vi "WriteBufferError.vi"(8 "error in (no error)":errorcluster, 11 "buffer-errors":T1 items=["No error"=0, "Generic Buffer error"=548500, "Generic Custom Buffer error"=548600, "Buffer is full"=548501, "Buffer is empty"=548502, "Buffer size cannot be 0"=548503, "Buffer reference is invalid"=548504, "Buffer event reference invalid"=548505, "Buffer Type not supported"=548506, "Not enough space in the buffer for this operation"=548507]) -> (0 "error out":errorcluster)   [LabVIEW 2013, in "CircularBuffer.lvlib" / "VariantBuffer.lvclass"]
uses:
  VariantBuffer.lvclass
  buffer-errors -- ring.ctl
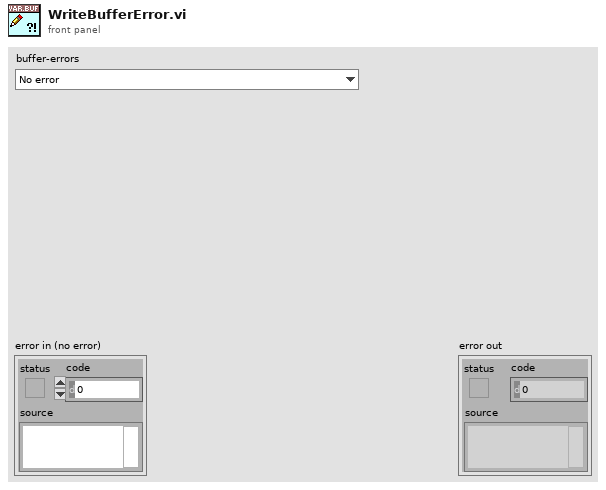
[diagram p1: front panel]
types:
  T1 = typedef "CircularBuffer.lvlib/VariantBuffer.lvclass/buffer-errors -- ring.ctl" = i32
  T2 = typedef "LVStringsAndValuesArrayTypeDef_I32.ctl" = cluster{"String":string, "Value":i32}[]
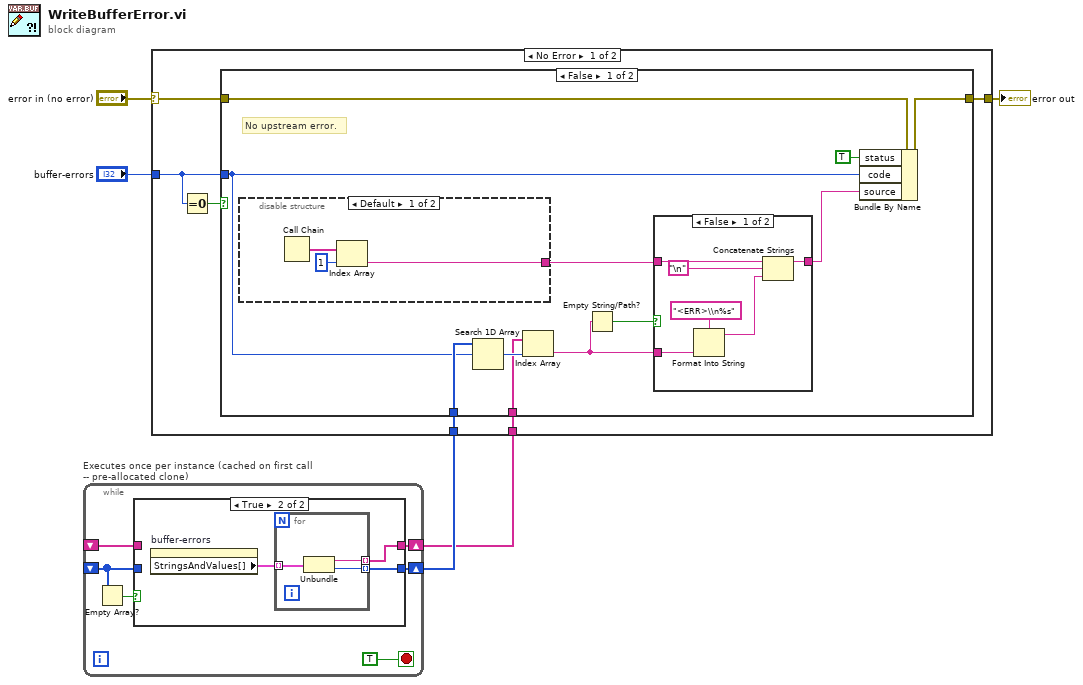
[diagram p0: block diagram]
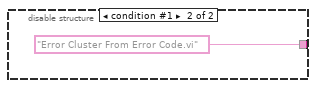
[diagram p4: hidden frame]
diagram:
  n1 = while "Executes once per instance (cached on first call -- pre-allocated clone)" {
    shift-right: [w11] -> w2
    shift-left: _ -> [w6]
    shift-right: [w10] -> w1
    shift-left: _ -> [w8]
    stop <- TRUE stop-if-true
    n2 = Empty Array?(array=w6) -> (empty?=w7:bool)
    n3 = case shown="True" w7 {
      tunnel: [w12 w15] -> w11
      tunnel: [w13 w14] -> w10
      tunnel: w6 -> [w12 _]
      tunnel: w8 -> [w13 _]
      frame False {
      }
      frame True {
        n4 = property on="buffer-errors" class="Ring (strict)"() -> ("StringsAndValues[]"=w16:T2)  [unwired: 2 in, 2 out]
        n5 = for {
          tunnel: w16 -> [w19] mode=indexing
          tunnel: [w18] -> w14 mode=indexing
          tunnel: [w17] -> w15 mode=indexing
          n6 = Unbundle(w19) -> ("String"=w18:string, "Value"=w17:i32)
        }
      }
    }
  }
  n7 = case shown="No Error" "error in (no error)" {
    selector: "error in (no error)" -> [w22 w49]
    tunnel: [w25 w49] -> w5
    tunnel: "buffer-errors" -> [w23 _]
    tunnel: w2 -> [w21 _]
    tunnel: w1 -> [w20 _]
    frame No Error {
      n8 = Equal To 0?(x=w23) -> (x = 0?=w24:bool)
      n9 = case shown="False" w24 {
        tunnel: w23 -> [w29 _]
        tunnel: w22 -> [w35 w48]
        tunnel: [w34 w48] -> w25
        tunnel: w21 -> [w30 _]
        tunnel: w20 -> [w27 _]
        frame False {
          # "No upstream error."
          n10 = disable-structure shown="Default" {
            disable-tunnel: [w44 "Error Cluster From Error Code.vi" ("source")] -> w32
            frame condition #0 (active) {
              n11 = Call Chain() -> (call chain=w45:string[])
              n12 = Index Array(array=w45, index=1) -> (element=w44:string)
            }
            frame condition #1 {
            }
          }
          n13 = Search 1D Array(1D array=w30, element=w29) -> (index of element=w28:i32)  [unwired: 1 in]
          n14 = Index Array(array=w27, index=w28) -> (element=w26:string)
          n15 = Empty String/Path?(string/path=w26) -> (empty?=w33:bool)
          n16 = case shown="False" w33 {
            tunnel: w26 -> [w38 _]
            tunnel: [w41 w43] -> w31
            tunnel: w32 -> [w42 w43]
            frame False {
              n17 = Format Into String(format string="<ERR>\\n%s", w38) -> (resulting string=w37:string)  [unwired: 2 in, 1 out]
              n18 = Concatenate Strings(w42, "\n", w37) -> (w41:string)
            }
            frame True {
            }
          }
          n19 = Bundle By Name(cluster=w35, "status"=TRUE, "code"=w29, "source"=w31) -> (w34:errorcluster)
        }
        frame True {
          # "Error code = 0, ignore"
        }
      }
    }
    frame Error {
      # "Upstream Error. Do not replace"
    }
  }
  "error out" <- w5
